vi "CODMn加标回收(子VI).vi"   [LabVIEW 2016, in "质控单元.lvlib"]
types:
  T1 = enum32{"Bad", "Idle", "Run top level", "Running"}
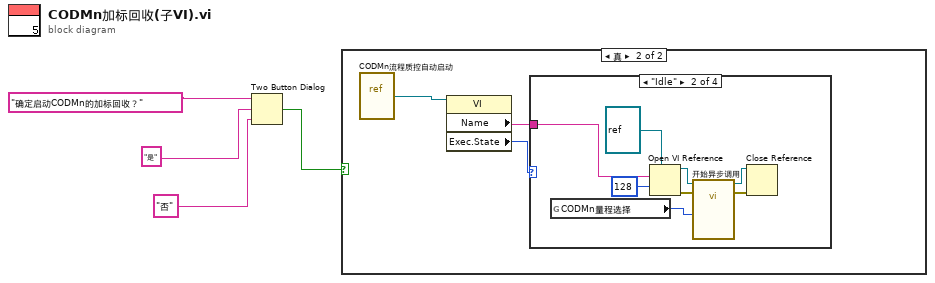
[diagram p0: block diagram]
diagram:
  n1 = Two Button Dialog(message="确定启动CODMn的加标回收？" ("消息"), 1:"否" ("F按钮名称（“取消”）"), 2:"是" ("T按钮名称（“确定”）")) -> (T button?=w4:bool)
  n2 = case shown="真" w4 {
    frame False {
    }
    frame True {
      n3 = vi-ref "CODMn流程质控自动启动.vi"() -> (w7:refnum<vi>)
      n4 = property class="VI"(reference=w7) -> ("Name"=w5:string, "Exec.State"=w6:T1)  [unwired: 1 in, 2 out]
      n5 = case shown="\"Idle\"" w6 {
        tunnel: w5 -> [_ w11 _ _]
        frame "Bad", Default {
        }
        frame "Idle" {
          n6 = global read "断电保存全局.vi" "CODMn量程选择"() -> (w8:enum32{"H", "L", "AUTO"})
          n7 = Open VI Reference(type specifier VI Refnum (for type only)=refnum<vi> refnum ("类型说明符VI引用句柄（仅用于类型）"), vi path=w11, options=128 ("选项")) -> (vi reference=w15:refnum<vi>, error out=w10:errorcluster)  [unwired: 3 in]
          n8 = call-by-ref "开始异步调用"(reference=w15, error in=w10, "CODMn量程切换"=w8) -> (reference out=w14:refnum<vi>, error out=w9:errorcluster)  [unwired: 10 in]
          n9 = Close Reference(reference=w14, error in (no error)=w9) -> ()  [unwired: 1 out]
        }
        frame "Run top level" {
        }
        frame "Running" {
        }
      }
    }
  }
